vi "Configure Contact Check.vi"(8 "error in (no error)":errorcluster, 9 "Contact Check On (T:On)":bool, 10 "Threshold  (2: OHM50)":u16(ring)=2 items=["OHM2", "OHM15", "OHM50"], 11 "VISA resource name":refnum<visa-resource-name>) -> (0 "error out":errorcluster, 3 "VISA resource name out":refnum<visa-resource-name>)   [LabVIEW 2020, in "Keithley 2450.lvlib"]
doc: "Use this command to enable or disable the contact check function.\n\n<B>The Digitizer Voltage and Digitizer Current functions are only compatible with the 2461.</B>"
uses:
  <instrlib>/Keithley 2450/Keithley 2450.lvlib
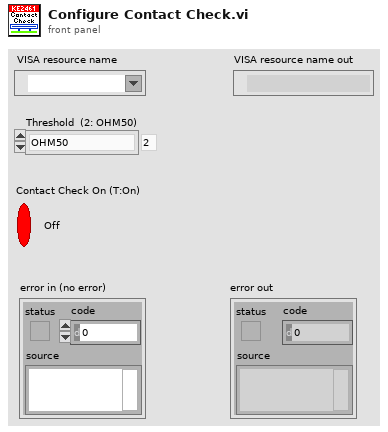
[diagram p1: front panel]
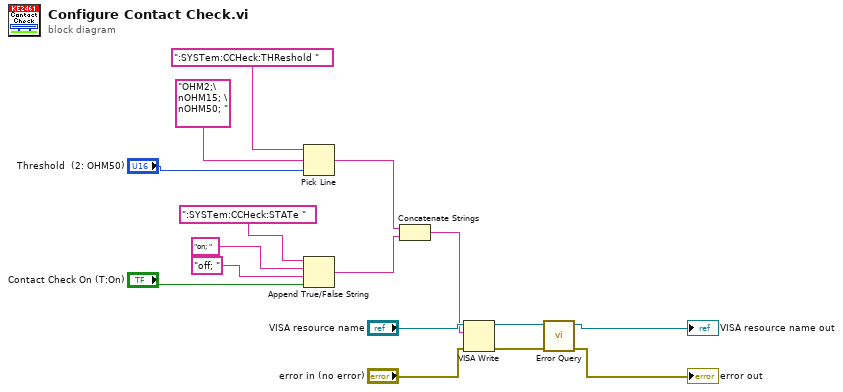
[diagram p0: block diagram]
diagram:
  n1 = Pick Line(string ("")=":SYSTem:CCHeck:THReshold ", multi-line string="OHM2;\nOHM15; \nOHM50; ", line index="Threshold  (2: OHM50)") -> (output string=w3:string)
  n2 = Append True/False String(1:"Contact Check On (T:On)", 2:"off; ", 3:"on; ", 4:":SYSTem:CCHeck:STATe ") -> (0:w2:string)
  n3 = Concatenate Strings(w3, w2) -> (w1:string)
  n4 = VISA Write(VISA resource name="VISA resource name", write buffer=w1, error in (no error)="error in (no error)") -> (VISA resource name out=w14:refnum<visa-resource-name>, error out=w13:errorcluster)  [unwired: 1 out]
  n5 = call <instrlib>:"Error Query.vi"("error in (no error)"=w13, "VISA resource name"=w14) -> ("error out"=→"error out":errorcluster, "VISA resource name out"=→"VISA resource name out":refnum<visa-resource-name>)  [unwired: 8 out]
